vi "Create RT FIFO.vi"(7 "fifo depth (10)":u32=10, 8 "error in (no error)":errorcluster, 11 "element size":u32 format="%d bytes") -> (0 "error out":errorcluster, 3 "rt fifo":refnum<k33>)   [LabVIEW 2021, in "DSF Core.lvlib" / "Interface.lvclass"]
uses:
  Interface.lvclass
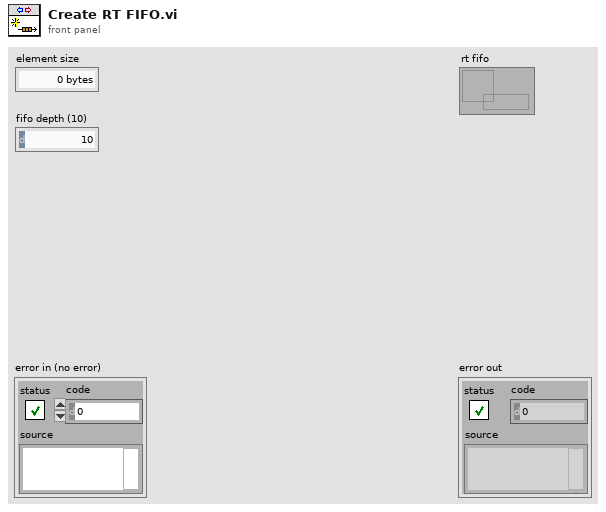
[diagram p1: front panel]
types:
  T1 = cluster{"read mode":enum16{"polling", "blocking"}, "write mode":enum16{"polling", "blocking"}}
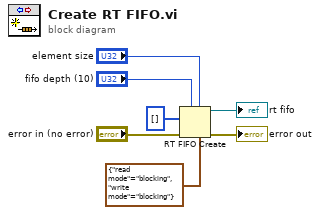
[diagram p0: block diagram]
diagram:
  n1 = RT FIFO Create(1:u8[] [], 3:"error in (no error)", 4:"fifo depth (10)", 6:"element size", 7:T1 {"read mode"=enum."blocking", "write mode"=enum."blocking"} ("r/w modes (polling,polling)")) -> (8:→"rt fifo":refnum<k33>, 11:→"error out":errorcluster)  [unwired: 3 in, 1 out]
